vi "Set_Post_Install_Step.vi"(8 "error in (no error)":errorcluster, 10 "data":T1, 11 "IB_Post_Install_Step in":refnum<class "IB_Post_Install_Step.lvclass">) -> (0 "error out":errorcluster, 3 "IB_Post_Install_Step out":refnum<class "IB_Post_Install_Step.lvclass">)   [LabVIEW 2020, in "IB_Post_Install_Step.lvclass"]
uses:
  <vilib>/AppBuilder/IB_Classes/Post_Install_Step/IB_Post_Install_Step.lvclass
  <vilib>/AppBuilder/IB_Classes/Post_Install_Step/IB_Post_Install_Step.lvclass/IB_Post_Install_Step.ctl
  <vilib>/AppBuilder/IB_Classes/Post_Install_Step/IB_Post_Install_Step.ctl
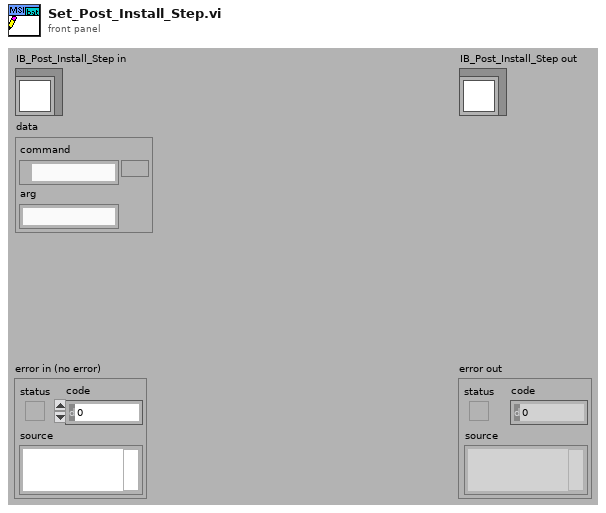
[diagram p1: front panel]
types:
  T1 = typedef "IB_Post_Install_Step.ctl" = cluster{"command":path, "arg":string}
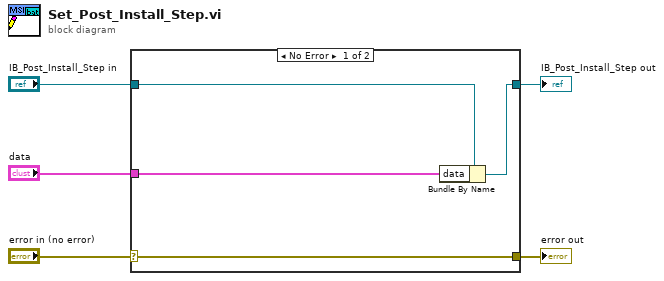
[diagram p0: block diagram]
diagram:
  n1 = case shown="No Error" "error in (no error)" {
    selector: "error in (no error)" -> [w9 w10]
    tunnel: [w9 w10] -> w4
    tunnel: [w7 w11] -> w2
    tunnel: "IB_Post_Install_Step in" -> [w8 w11]
    tunnel: "data" -> [w6 _]
    frame No Error {
      n2 = Bundle By Name(cluster=w8, "data"=w6) -> (w7:refnum<class "IB_Post_Install_Step.lvclass">)
    }
    frame Error {
    }
  }
  "error out" <- w4
  "IB_Post_Install_Step out" <- w2
